vi "Reset.vi"(8 "error in (no error)":errorcluster, 11 "Ticker in":refnum<class "Ticker.lvclass">) -> (0 "error out":errorcluster, 3 "Ticker out":refnum<class "Ticker.lvclass">)   [LabVIEW 2013, in "Ticker.lvclass"]
uses:
  Ticker.lvclass
  Ticker.lvclass/Ticker.ctl
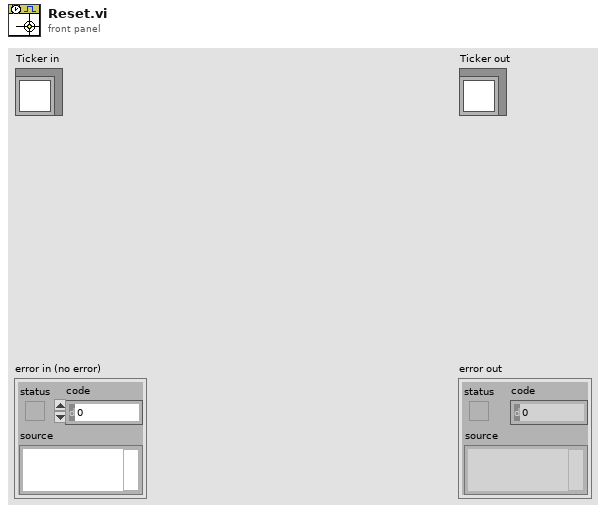
[diagram p1: front panel]
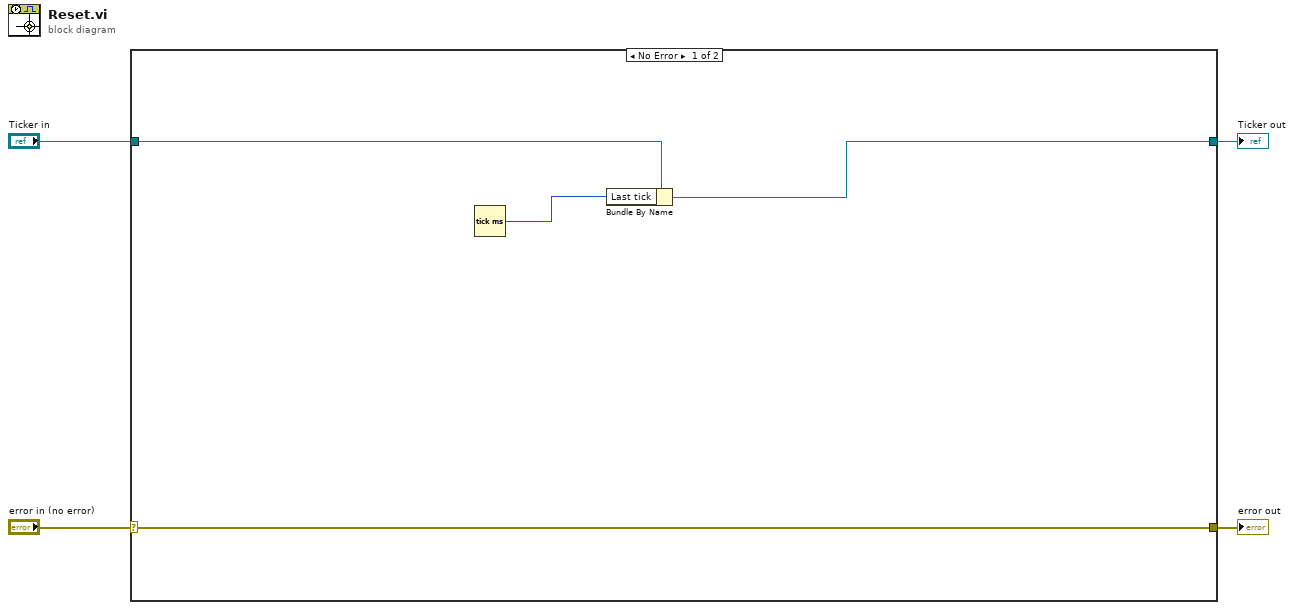
[diagram p0: block diagram]
diagram:
  n1 = case shown="No Error" "error in (no error)" {
    selector: "error in (no error)" -> [w8 w10]
    tunnel: [w8 w10] -> w3
    tunnel: [w5 w9] -> w1
    tunnel: "Ticker in" -> [w6 w9]
    frame No Error {
      n2 = Tick Count (ms)() -> (millisecond timer value=w7:u32)
      n3 = Bundle By Name(cluster=w6, "Last tick"=w7) -> (w5:refnum<class "Ticker.lvclass">)
    }
    frame Error {
    }
  }
  "error out" <- w3
  "Ticker out" <- w1
